vi "Won.vi"(8 "error in (no error)":errorcluster, 10 "Num Targets":i32, 11 "Player in":refnum<class "Player.lvclass">) -> (0 "error out":errorcluster, 2 "Won?":bool, 3 "Player out":refnum<class "Player.lvclass">)   [LabVIEW 2015, in "Player.lvclass"]
uses:
  Player.lvclass
  Player.lvclass/Player.ctl
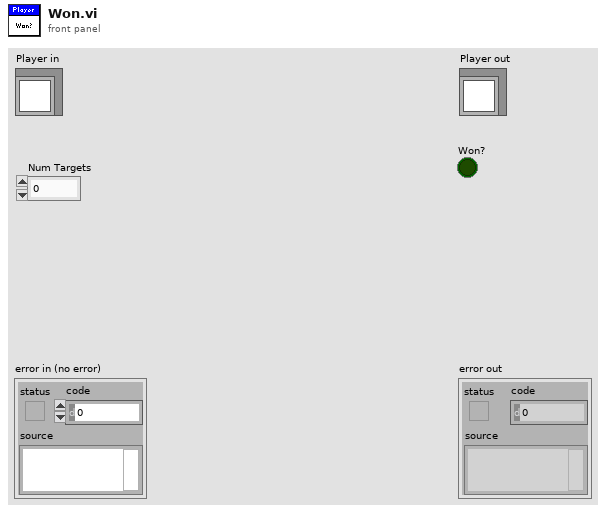
[diagram p1: front panel]
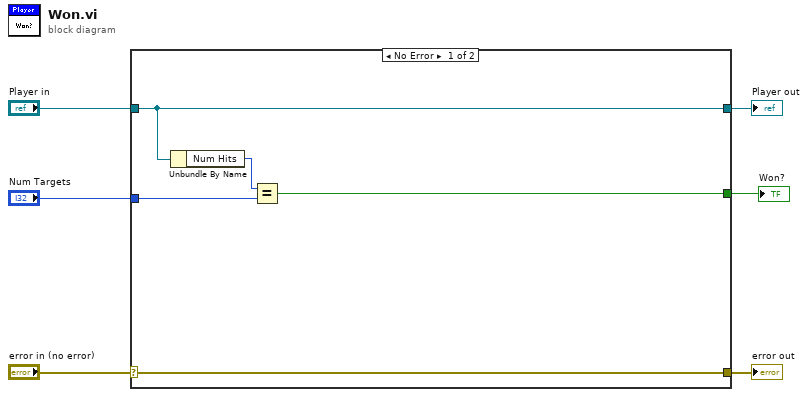
[diagram p0: block diagram]
diagram:
  n1 = case shown="No Error" "error in (no error)" {
    selector: "error in (no error)" -> [w11 w13]
    tunnel: [w11 w13] -> w5
    tunnel: [w10 w12] -> w3
    tunnel: "Player in" -> [w10 w12]
    tunnel: "Num Targets" -> [w8 _]
    tunnel: [w7 _] -> w1
    frame No Error {
      n2 = Unbundle By Name(w10) -> ("Num Hits"=w9:i32)
      n3 = Equal?(x=w9, y=w8) -> (x = y?=w7:bool)
    }
    frame Error {
    }
  }
  "error out" <- w5
  "Player out" <- w3
  "Won?" <- w1
